vi "Started.vi"(8 "error in (no error)":errorcluster, 11 "Command State Actor in":refnum<class "Command State Actor.lvclass">) -> (0 "error out":errorcluster, 3 "Command State Actor out":refnum<class "Command State Actor.lvclass">)   [LabVIEW 2013, in "Command State Actor.lvlib" / "Command State Actor.lvclass"]
uses:
  Command State Actor.lvclass
  Command States.ctl
  <vilib>/ActorFramework/Actor/Actor.lvclass/Actor.ctl
  <vilib>/ActorFramework/Message Enqueuer/Message Enqueuer.lvclass/Message Enqueuer.ctl
  <vilib>/ActorFramework/Message Enqueuer/Init from Existing Queue.vi
  <vilib>/ActorFramework/Message Enqueuer/Enqueue.vi
  <vilib>/ActorFramework/Message Priority Queue/Priority Enqueue.vi
  <vilib>/ActorFramework/Message Enqueuer/Message Enqueuer.lvclass
  Command State Actor Messages/Go To Executing Msg/Go To Executing Msg.lvclass
  <vilib>/ActorFramework/Actor/Actor.lvclass
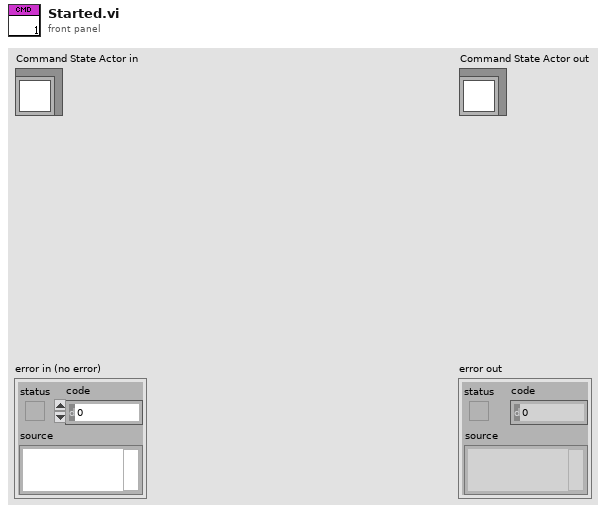
[diagram p1: front panel]
types:
  T1 = typedef "Command State Actor.lvlib/Command State Actor.lvclass/Command States.ctl" = enum16{"NotStarted", "Starting", "Started", "Executing", "Completing", "Completed", "Stopping", "Stopped"}
  T2 = typedef "Command State Actor.lvlib/Command State Actor.lvclass/Command Status.ctl" = cluster{"CurrentCommandState":T1, "Command Name":string, "Current State Status":T3, "Command Start Time":timestamp, "Command End Time":timestamp, "Previous State Status":T3}
  T3 = typedef "Command Actor.lvlib/Command States.lvclass/State Status.ctl" = cluster{"State Name":string, "State Entry Time":timestamp, "State Exit Time":timestamp}
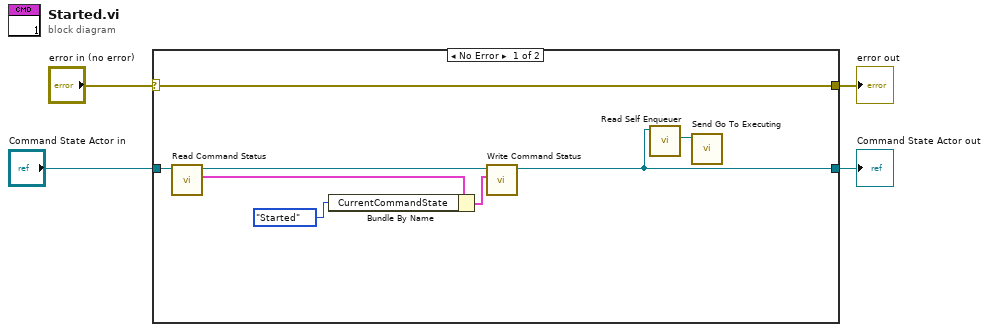
[diagram p0: block diagram]
diagram:
  n1 = case shown="No Error" "error in (no error)" {
    selector: "error in (no error)" -> [w12 w14]
    tunnel: [w12 w14] -> w3
    tunnel: [w6 w13] -> w1
    tunnel: "Command State Actor in" -> [w11 w13]
    frame No Error {
      n2 = call-dynamic "Read Command Status.vi"("Command in"=w11) -> ("Command Status"=w9:T2, "Command out"=w10:refnum<class "Command State Actor.lvclass">)  [unwired: 8 in, 1 out]
      n3 = Bundle By Name(cluster=w9, "CurrentCommandState"=Command_States."Started") -> (w8:T2)
      n4 = call-dynamic "Write Command Status.vi"("Command Status"=w8, "Command in"=w10) -> ("Command out"=w6:refnum<class "Command State Actor.lvclass">)  [unwired: 8 in, 1 out]
      n5 = call <vilib>:"Read Self Enqueuer.vi"("Actor"=w6) -> ("Self Enqueuer"=w5:refnum<class "Message Enqueuer.lvclass">)  [unwired: 10 in]
      n6 = call "Send Go To Executing.vi"("Message Enqueuer"=w5) -> ()  [unwired: 9 in, 2 out]
    }
    frame Error {
    }
  }
  "error out" <- w3
  "Command State Actor out" <- w1
